vi "drive shooting normalizer.vi"(1 "input":dbl) -> (0 "output":dbl)   [LabVIEW 2011]
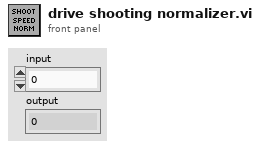
[diagram p1: front panel]
types:
  T1 = typedef "WPI_EncoderDevRef.ctl" = cluster{"DevStatus":errorcluster, "EncoderIndex":T2, "CounterIndex":T3, "DistancePerCount":dbl, "Decoding Type":T4}
  T2 = typedef "FPGA_EncoderIdx.ctl" = enum8{"Enc 0", "Enc 1", "Enc 2", "Enc 3", "Invalid"}
  T3 = typedef "FPGA_CounterCtrSystemIndex.ctl" = enum8{"Ctr 0", "Ctr 1", "Ctr 2", "Ctr 3", "Ctr 4", "Ctr 5", "Ctr 6", "Ctr 7", "Invalid"}
  T4 = typedef "WPI_EncoderType.ctl" = enum16{"1x", "2x", "4x"}
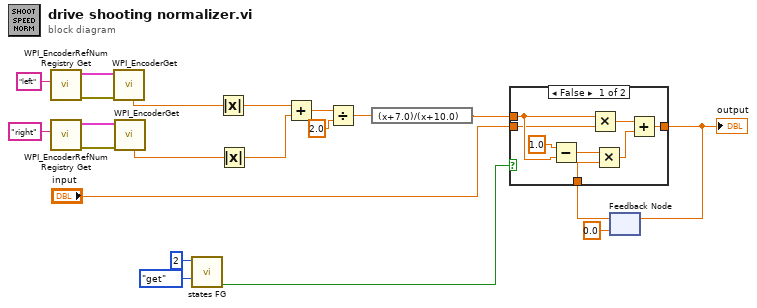
[diagram p0: block diagram]
diagram:
  n1 = call <vilib>:"WPI_EncoderRefNum Registry Get.vi"("refnum name"="left") -> ("error out"=w17:errorcluster, "EncoderDevRef"=w19:T1)  [unwired: 9 in]
  n2 = call <vilib>:"WPI_EncoderRefNum Registry Get.vi"("refnum name"="right") -> ("error out"=w16:errorcluster, "EncoderDevRef"=w18:T1)  [unwired: 9 in]
  n3 = call <vilib>:"WPI_EncoderGet.vi"("error in (no error)"=w17, "EncoderDevRef"=w19) -> ("Rate"=w11:dbl)  [unwired: 4 in, 5 out]
  n4 = call <vilib>:"WPI_EncoderGet.vi"("error in (no error)"=w16, "EncoderDevRef"=w18) -> ("Rate"=w10:dbl)  [unwired: 4 in, 5 out]
  n5 = call "states FG.vi"("menu (get)"=enum16{"set", "get"}."get", "Loop ID"=2) -> ("first call?"=w1:bool)  [unwired: 6 in, 3 out]
  n6 = Absolute Value(x=w11) -> (abs(x)=w14:dbl)
  n7 = Absolute Value(x=w10) -> (abs(x)=w15:dbl)
  n8 = Add(x=w14, y=w15) -> (x+y=w12:dbl)
  n9 = Divide(x=w12, y=2.0) -> (x/y=w9:dbl)
  n10 = expression code="(x+7.0)/(x+10.0)"(w9) -> (w8:dbl)
  n11 = feedback #1(0.0) -> (w6:dbl)
  n12 = case shown="False" w1 {
    tunnel: w8 -> [w25 _]
    tunnel: [w24 w30] -> w7
    tunnel: w6 -> [w23 _]
    tunnel: "input" -> [w22 w30]
    frame False {
      n13 = Subtract(x=1.0, y=w25) -> (x-y=w27:dbl)
      n14 = Multiply(x=w25, y=w22) -> (x*y=w29:dbl)
      n15 = Multiply(x=w27, y=w23) -> (x*y=w28:dbl)
      n16 = Add(x=w29, y=w28) -> (x+y=w24:dbl)
    }
    frame True {
    }
  }
  "output" <- w7
  n17 = feedback-in #1(w7) -> ()
